vi "Pfeiffer-RVC300.ProcEvents.vi"(0 "i ref in":refnum<vi>, 5 "error in":errorcluster) -> (14 "i ref out":refnum<vi>, 19 "error out":errorcluster)   [LabVIEW 2014, in "Pfeiffer-RVC300.lvlib"]
doc: "This method is used to define the events the object will listen to. Add your own events here."
uses:
  Pfeiffer-RVC300.lvlib
  CS_Core/BaseProcess/BaseProcess.event definition.ctl
  CS_Core/CAEObj/CAEObj.event definition.ctl
  CS_Core/BaseProcess/BaseProcess.descriptor string definition.ctl
  CS_Core/BaseProcess/BaseProcess.lvlib
  CS_Core/CAEObj/CAEObj.lvlib
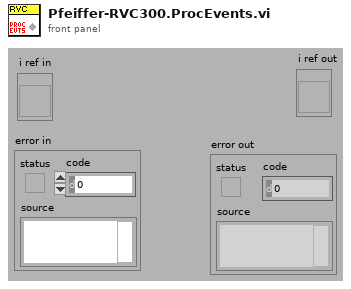
[diagram p1: front panel]
types:
  T1 = typedef "BaseProcess.lvlib/BaseProcess.event definition.ctl" = cluster{"CAEEvtDef":T2, "Data Descriptor":T3}
  T2 = typedef "CAEObj.lvlib/CAEObj.event definition.ctl" = cluster{"URL":string, "enable":bool, "ignoreResID":bool}
  T3 = typedef "BaseProcess.lvlib/BaseProcess.descriptor string definition.ctl" = string
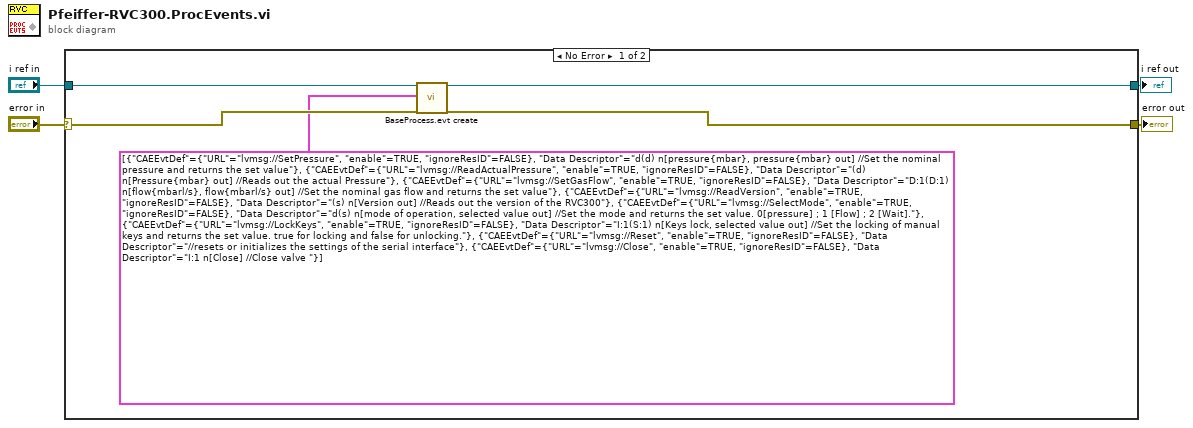
[diagram p0: block diagram]
diagram:
  n1 = case shown="No Error" "error in" {
    selector: "error in" -> [w6 w10]
    tunnel: "i ref in" -> [w9 w11]
    tunnel: [w8 w11] -> w3
    tunnel: [w7 w10] -> w2
    frame No Error {
      n2 = call "BaseProcess.evt create.vi"("i ref in"=w9, "newEvents"=T1[] [{"CAEEvtDef"={"URL"="lvmsg://SetPressure", "enable"=TRUE, "ignoreResID"=FALSE}, "Data Descriptor"="d(d) n[pressure{mbar}, pressure{mbar} out] //Set the nominal pressure and returns the set value"}, {"CAEEvtDef"={"URL"="lvmsg://ReadActualPressure", "enable"=TRUE, "ignoreResID"=FALSE}, "Data Descriptor"="(d) n[Pressure{mbar} out] //Reads out the actual Pressure"}, {"CAEEvtDef"={"URL"="lvmsg://SetGasFlow", "enable"=TRUE, "ignoreResID"=FALSE}, "Data Descriptor"="D:1(D:1) n[flow{mbarl/s}, flow{mbarl/s} out] //Set the nominal gas flow and returns the set value"}, {"CAEEvtDef"={"URL"="lvmsg://ReadVersion", "enable"=TRUE, "ignoreResID"=FALSE}, "Data Descriptor"="(s) n[Version out] //Reads out the version of the RVC300"}, {"CAEEvtDef"={"URL"="lvmsg://SelectMode", "enable"=TRUE, "ignoreResID"=FALSE}, "Data Descriptor"="d(s) n[mode of operation, selected value out] //Set the mode and returns the set value. 0[pressure] ; 1 [Flow] ; 2 [Wait]."}, {"CAEEvtDef"={"URL"="lvmsg://LockKeys", "enable"=TRUE, "ignoreResID"=FALSE}, "Data Descriptor"="I:1(S:1) n[Keys lock, selected value out] //Set the locking of manual keys and returns the set value. true for locking and false for unlocking."}, {"CAEEvtDef"={"URL"="lvmsg://Reset", "enable"=TRUE, "ignoreResID"=FALSE}, "Data Descriptor"="//resets or initializes the settings of the serial interface"}, {"CAEEvtDef"={"URL"="lvmsg://Close", "enable"=TRUE, "ignoreResID"=FALSE}, "Data Descriptor"="I:1 n[Close] //Close valve "}] ("new events"), "error in (no error)"=w6) -> ("i ref out"=w8:refnum<vi>, "error out"=w7:errorcluster)  [unwired: 13 in, 2 out]
    }
    frame Error {
    }
  }
  "i ref out" <- w3
  "error out" <- w2
